vi "DHE_VAR_DACsFile.vi"(9 "value":path, 10 "action":T1) -> (1 "DacFilePath":path)   [LabVIEW 2016]
uses:
  DHE_VarAction.ctl
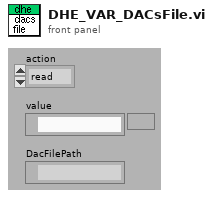
[diagram p1: front panel]
types:
  T1 = typedef "DHE_VarAction.ctl" = enum16{"read", "write"}
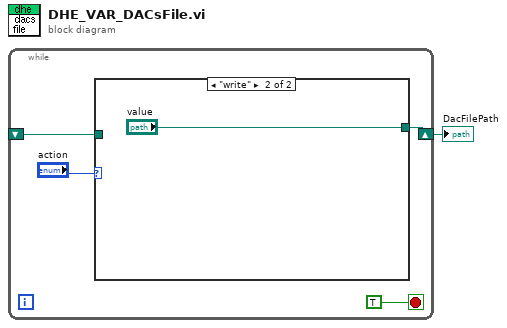
[diagram p0: block diagram]
diagram:
  n1 = while {
    shift-right: [w4] -> w1
    shift-left: _ -> [w3]
    stop <- TRUE stop-if-true
    n2 = case shown="\"write\"" "action" {
      tunnel: [w6 "value"] -> w4
      tunnel: w3 -> [w6 _]
      frame "read", Default {
      }
      frame "write" {
      }
    }
  }
  "DacFilePath" <- w1
